vi "VCS Get Ipm Status.vi"(6 "error in (no error)":errorcluster, 9 "axis in":cluster{"keyHandle":u32, "nodeId":u16}={"keyHandle"=0, "nodeId"=1}) -> (0 "error out":errorcluster, 2 "IPM status":T1, 3 "axis out":cluster{"keyHandle":u32, "nodeId":u16}={"keyHandle"=0, "nodeId"=1})   [LabVIEW 2019, in "maxonEPOS.lvlib"]
doc: "The function <B>VCS_GetIpmStatus</B> returns all IPM warning and error states."
uses:
  Examples/maxonEPOS.lvlib
  Resources/EposCmd.dll
  Resources/EposCmd64.dll
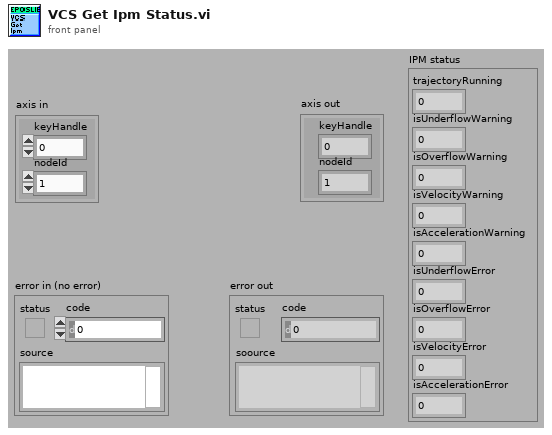
[diagram p1: front panel]
types:
  T1 = cluster{"trajectoryRunning":i32, "isUnderflowWarning":i32, "isOverflowWarning":i32, "isVelocityWarning":i32, "isAccelerationWarning":i32, "isUnderflowError":i32, "isOverflowError":i32, "isVelocityError":i32, "isAccelerationError":i32}
  T2 = cluster{"pSpeedIndex 3":u32, "pHomePosition":i32, i32, "pSpeedSwitch":u32, "pSpeedIndex":u32, "pHomingAcceleration":u32, "pCurrentThreshold":u16, "pHomeOffset":i32, "pSpeedIndex 2":u32}
  T3 = cluster{"pTrajectoryRunning":i32, "pIsUnderflowWarning":i32, "pIsOverflowWarning":i32, "pIsVelocityWarning":i32, "pIsAccelerationWarning":i32, "pIsUnderflowError":i32, "pIsOverflowError":i32, "pIsVelocityError":i32, "pIsAccelerationError":i32}
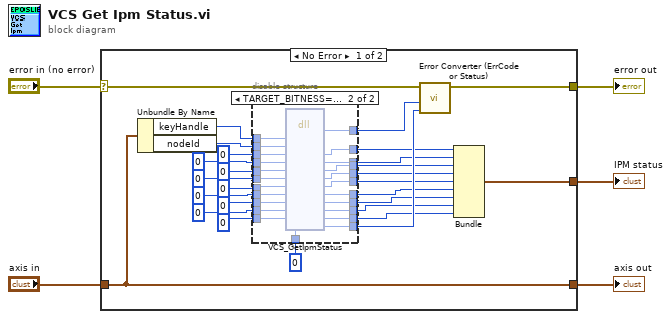
[diagram p0: block diagram]
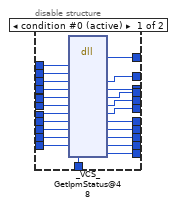
[diagram p2: hidden frame]
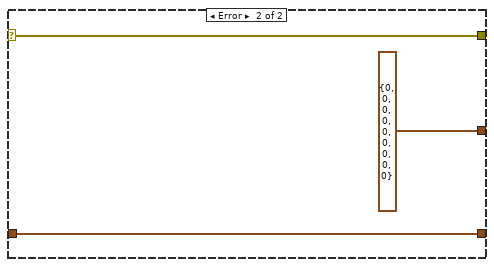
[diagram p3: hidden frame]
diagram:
  n1 = case shown="No Error" "error in (no error)" {
    selector: "error in (no error)" -> [w30 w80]
    tunnel: "axis in" -> [w32 w81]
    tunnel: [w32 w81] -> w4
    tunnel: [w31 w80] -> w3
    tunnel: [w8 T2 {"pSpeedIndex 3"=0, "pHomePosition"=0, 0, "pSpeedSwitch"=0, "pSpeedIndex"=0, "pHomingAcceleration"=0, "pCurrentThreshold"=0, "pHomeOffset"=0, "pSpeedIndex 2"=0}] -> w1
    frame No Error {
      n2 = Unbundle By Name(w32) -> ("keyHandle"=w27:u32, "nodeId"=w28:u16)
      n3 = disable-structure shown="TARGET_BITNESS==64" {
        disable-tunnel: u32 0 ("pErrorCode") -> [w55 w78]
        disable-tunnel: w28 -> [w54 w77]
        disable-tunnel: w27 -> [w53 w76]
        disable-tunnel: [w52 w75] -> w26
        disable-tunnel: [w51 w74] -> w25
        disable-tunnel: 0 ("pTrajectoryRunning") -> [w50 w73]
        disable-tunnel: 0 ("pIsUnderflowWarning") -> [w49 w72]
        disable-tunnel: 0 ("pIsAccelerationWarning") -> [w48 w71]
        disable-tunnel: 0 ("pIsVelocityWarning") -> [w47 w70]
        disable-tunnel: 0 ("pIsAccelerationError") -> [w46 w69]
        disable-tunnel: 0 ("pIsVelocityError") -> [w45 w68]
        disable-tunnel: 0 ("pIsOverflowError") -> [w44 w67]
        disable-tunnel: [w43 w66] -> w17
        disable-tunnel: [w42 w65] -> w16
        disable-tunnel: [w41 w64] -> w15
        disable-tunnel: [w40 w63] -> w14
        disable-tunnel: [w39 w62] -> w13
        disable-tunnel: [w38 w61] -> w12
        disable-tunnel: [w37 w60] -> w11
        disable-tunnel: [w36 w59] -> w10
        disable-tunnel: [w35 w58] -> w9
        disable-tunnel: 0 ("pIsOverflowWarning") -> [w34 w57]
        disable-tunnel: 0 ("pIsUnderflowError") -> [w33 w56]
        frame condition #0 (active) {
          n4 = dll-call lib="C:/workspace/project/scancon/sw/SSI_Tool/InstrumentsInterfaces/Motordriver/maxon EPOS/Resources/EposCmd.*" fn="_VCS_GetIpmStatus@48"("KeyHandle"=w53, "NodeId"=w54, "pTrajectoryRunning"=w50, "pIsUnderflowWarning"=w49, "pIsOverflowWarning"=w34, "pIsVelocityWarning"=w47, "pIsAccelerationWarning"=w48, "pIsUnderflowError"=w33, "pIsOverflowError"=w44, "pIsVelocityError"=w45, "pIsAccelerationError"=w46, "pErrorCode"=w55) -> (w52:i32, "pTrajectoryRunning"=w43:i32, "pIsUnderflowWarning"=w42:i32, "pIsOverflowWarning"=w41:i32, "pIsVelocityWarning"=w40:i32, "pIsAccelerationWarning"=w39:i32, "pIsUnderflowError"=w38:i32, "pIsOverflowError"=w37:i32, "pIsVelocityError"=w36:i32, "pIsAccelerationError"=w35:i32, "pErrorCode"=w51:u32)  [unwired: 5 in, 2 out]
        }
        frame condition #1 {
          n5 = dll-call lib="C:/Sources/LabView/maxon EPOS/Resources/EposCmd64.*" fn="VCS_GetIpmStatus" ("EposCmd.dll:_VCS_GetIpmStatus@48")("KeyHandle"=w76, "NodeId"=w77, "pTrajectoryRunning"=w73, "pIsUnderflowWarning"=w72, "pIsOverflowWarning"=w57, "pIsVelocityWarning"=w70, "pIsAccelerationWarning"=w71, "pIsUnderflowError"=w56, "pIsOverflowError"=w67, "pIsVelocityError"=w68, "pIsAccelerationError"=w69, "pErrorCode"=w78) -> ("Rückgabetyp"=w75:i32, "pTrajectoryRunning"=w66:i32, "pIsUnderflowWarning"=w65:i32, "pIsOverflowWarning"=w64:i32, "pIsVelocityWarning"=w63:i32, "pIsAccelerationWarning"=w62:i32, "pIsUnderflowError"=w61:i32, "pIsOverflowError"=w60:i32, "pIsVelocityError"=w59:i32, "pIsAccelerationError"=w58:i32, "pErrorCode"=w74:u32)  [unwired: 5 in, 2 out]
        }
      }
      n6 = call "Error Converter (ErrCode or Status).vi"("error code"=w25, "return type"=w26, "error in (no error)"=w30) -> ("error out"=w31:errorcluster)  [unwired: 7 in]
      n7 = Bundle("pTrajectoryRunning"=w17, "pIsUnderflowWarning"=w16, "pIsOverflowWarning"=w15, "pIsVelocityWarning"=w14, "pIsAccelerationWarning"=w13, "pIsUnderflowError"=w12, "pIsOverflowError"=w11, "pIsVelocityError"=w10, "pIsAccelerationError"=w9) -> (w8:T3)  [unwired: 1 in]
    }
    frame Error {
    }
  }
  "error out" <- w3
  "axis out" <- w4
  "IPM status" <- w1
